vi "S2DS_ConfigWrite sweep info (SubVI).vi"(8 "error in (no error)":errorcluster, 9 "WC Channel names":string[](array[string]), 10 "Scan parameters in":T2 {"Y data taking" items=["in both direction", "in up direction only", "in down direction only"]; "X data taking" items=["in both direction", "in up direction only", "in down direction only"]}, 11 "Refnum in":T1) -> (0 "error out":errorcluster, 3 "Refnum out":T1)   [LabVIEW 2025]
uses:
  TYPE DEFS/S2DS_Sweep Info.ctl
  <vilib>/Utility/config.llb/Config Data RefNum.ctl
  <vilib>/Utility/config.llb/Write Key (String).vi
  <vilib>/Utility/config.llb/Write Key (I32).vi
  <vilib>/Utility/config.llb/Write Key (Double).vi
  <vilib>/Utility/config.llb/Write Key (U32).vi
  <vilib>/Utility/config.llb/Write Key (Boolean).vi
  <vilib>/Utility/config.llb/NI_LVConfig.lvlib
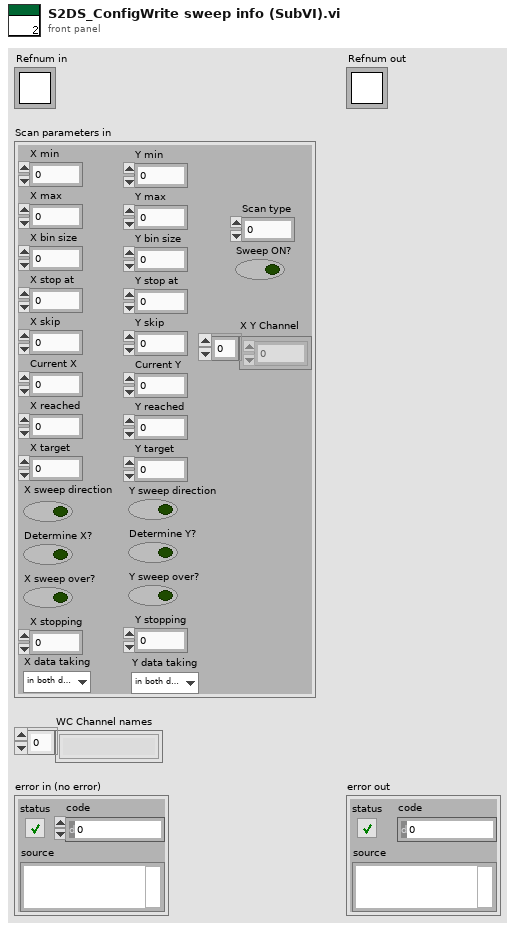
[diagram p1: front panel]
types:
  T1 = typedef "NI_LVConfig.lvlib/Config Data RefNum.ctl" = refnum<k1>
  T2 = typedef "S2DS_Sweep Info.ctl" = cluster{"X min":ext, "X max":dbl, "Y min":dbl, "Y max":dbl, "X bin size":dbl, "Y bin size":dbl, "X stop at":dbl, "Y stop at":dbl, "X skip":u64, "Y skip":u64, "Current X":dbl, "Current Y":dbl, "X reached":i32, "Y reached":i32, "X target":dbl, "Y target":dbl, "Sweep ON?":bool, "X sweep direction":bool, "Y sweep direction":bool, "Determine X?":bool, "Determine Y?":bool, "X sweep over?":bool, "Y sweep over?":bool, "Scan type":i32, "X stopping":i32, "Y stopping":i32, "X Y Channel":u16[], "X data taking":u16, "Y data taking":u16}
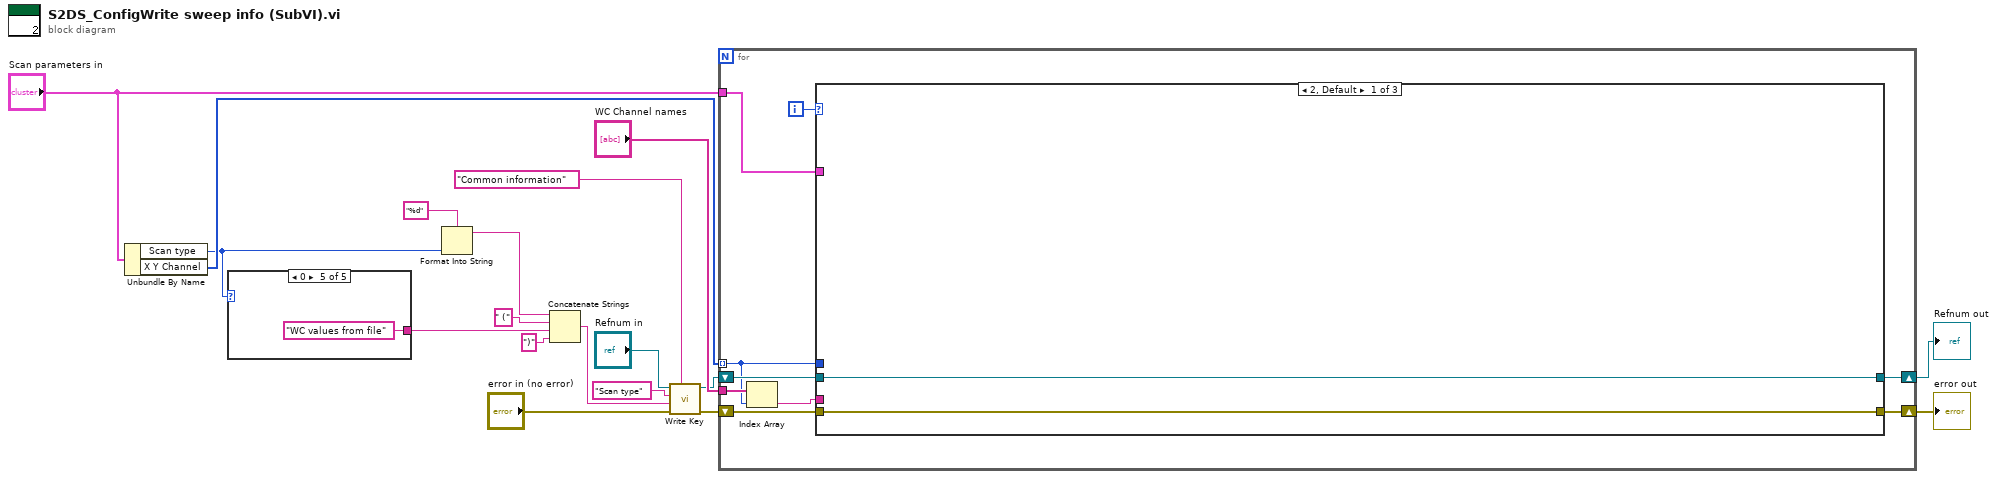
[diagram p0: block diagram]
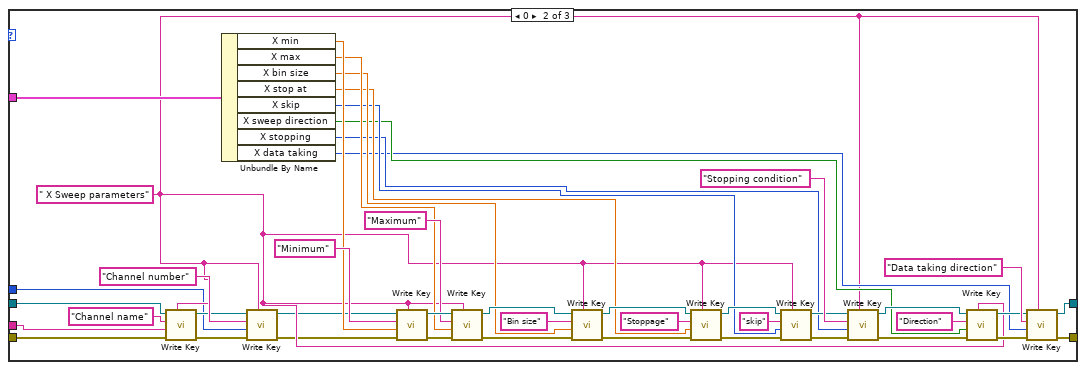
[diagram p2: hidden frame]
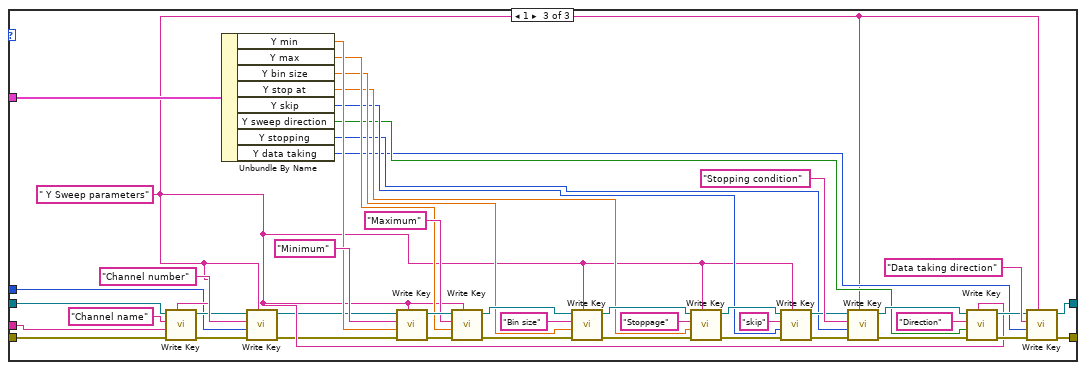
[diagram p3: hidden frame]
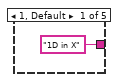
[diagram p4: hidden frame]
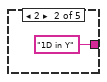
[diagram p5: hidden frame]
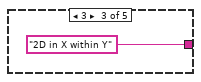
[diagram p6: hidden frame]
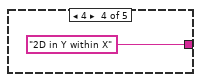
[diagram p7: hidden frame]
diagram:
  n1 = Unbundle By Name("Scan parameters in") -> ("Scan type"=w7:i32, "X Y Channel"=w10:u16[])
  n2 = case shown="0" w7 {
    tunnel: ["1D in X" "1D in Y" "2D in X within Y" "2D in Y within X" "WC values from file"] -> w2
    frame 1, Default {
    }
    frame 2 {
    }
    frame 3 {
    }
    frame 4 {
    }
    frame 0 {
    }
  }
  n3 = Format Into String(format string="%d", w7) -> (resulting string=w5:string)  [unwired: 2 in, 1 out]
  n4 = Concatenate Strings(w5, " (" ("string"), w2, ")" ("string")) -> (w1:string)
  n5 = call-poly <vilib>:"Write Key.vi"("section"="Common information", "error in (no error)"="error in (no error)", "value"=w1, "key"="Scan type", "refnum"="Refnum in") -> ("error out"=w12:errorcluster, "refnum out"=w11:T1)  [unwired: 4 in, 1 out]
  n6 = for {
    tunnel: w10 -> [w24] mode=indexing
    tunnel: "WC Channel names" -> [w32]
    shift-right: [w28] -> w14
    shift-left: w11 -> [w29]
    shift-right: [w27] -> w15
    shift-left: w12 -> [w30]
    tunnel: "Scan parameters in" -> [w31]
    i -> [w26]
    n7 = Index Array(array=w32, index=w24) -> (element=w25:string)
    n8 = case shown="2, Default" w26 {
      tunnel: w31 -> [_ w71 w115]
      tunnel: [w34 w47 w91] -> w28
      tunnel: [w33 w48 w92] -> w27
      tunnel: w29 -> [w34 w38 w82]
      tunnel: w30 -> [w33 w36 w80]
      tunnel: w25 -> [_ w44 w88]
      tunnel: w24 -> [_ w39 w83]
      frame 2, Default {
      }
      frame 0 {
        w41 = " X Sweep parameters"
        n9 = call-poly <vilib>:"Write Key.vi"("section"=w41, "error in (no error)"=w36, "value"=w44, "key"="Channel name", "refnum"=w38) -> ("error out"=w40:errorcluster, "refnum out"=w42:T1)  [unwired: 4 in, 1 out]
        n10 = Unbundle By Name(w71) -> ("X min"=w70:ext, "X max"=w69:dbl, "X bin size"=w68:dbl, "X stop at"=w55:dbl, "X skip"=w54:u64, "X sweep direction"=w53:bool, "X stopping"=w52:i32, "X data taking"=w46:u16)
        n11 = call-poly <vilib>:"Write Key.vi"("section"=w41, "error in (no error)"=w40, "value"=w39, "key"="Channel number", "refnum"=w42) -> ("error out"=w35:errorcluster, "refnum out"=w37:T1)  [unwired: 4 in, 1 out]
        n12 = call-poly <vilib>:"Write Key.vi"("section"=w41, "error in (no error)"=w35, "value"=w70, "key"="Minimum", "refnum"=w37) -> ("error out"=w77:errorcluster, "refnum out"=w75:T1)  [unwired: 4 in, 1 out]
        n13 = call-poly <vilib>:"Write Key.vi"("section"=w41, "error in (no error)"=w77, "value"=w69, "key"="Maximum", "refnum"=w75) -> ("error out"=w78:errorcluster, "refnum out"=w76:T1)  [unwired: 4 in, 1 out]
        n14 = call-poly <vilib>:"Write Key.vi"("section"=w41, "error in (no error)"=w78, "value"=w68, "key"="Bin size", "refnum"=w76) -> ("error out"=w56:errorcluster, "refnum out"=w57:T1)  [unwired: 4 in, 1 out]
        n15 = call-poly <vilib>:"Write Key.vi"("section"=w41, "error in (no error)"=w56, "value"=w55, "key"="Stoppage", "refnum"=w57) -> ("error out"=w60:errorcluster, "refnum out"=w63:T1)  [unwired: 4 in, 1 out]
        n16 = call-poly <vilib>:"Write Key.vi"("section"=w41, "error in (no error)"=w60, "value"=w54, "key"="skip", "refnum"=w63) -> ("error out"=w59:errorcluster, "refnum out"=w62:T1)  [unwired: 4 in, 1 out]
        n17 = call-poly <vilib>:"Write Key.vi"("section"=w41, "error in (no error)"=w59, "value"=w52, "key"="Stopping condition", "refnum"=w62) -> ("error out"=w58:errorcluster, "refnum out"=w61:T1)  [unwired: 4 in, 1 out]
        n18 = call-poly <vilib>:"Write Key.vi"("section"=w41, "error in (no error)"=w58, "value"=w53, "key"="Direction", "refnum"=w61) -> ("error out"=w49:errorcluster, "refnum out"=w50:T1)  [unwired: 4 in, 1 out]
        n19 = call-poly <vilib>:"Write Key.vi"("section"=w41, "error in (no error)"=w49, "value"=w46, "key"="Data taking direction", "refnum"=w50) -> ("error out"=w48:errorcluster, "refnum out"=w47:T1)  [unwired: 4 in, 1 out]
      }
      frame 1 {
        w85 = " Y Sweep parameters"
        n20 = call-poly <vilib>:"Write Key.vi"("section"=w85, "error in (no error)"=w80, "value"=w88, "key"="Channel name", "refnum"=w82) -> ("error out"=w84:errorcluster, "refnum out"=w86:T1)  [unwired: 4 in, 1 out]
        n21 = Unbundle By Name(w115) -> ("Y min"=w114:dbl, "Y max"=w113:dbl, "Y bin size"=w112:dbl, "Y stop at"=w99:dbl, "Y skip"=w98:u64, "Y sweep direction"=w97:bool, "Y stopping"=w96:i32, "Y data taking"=w90:u16)
        n22 = call-poly <vilib>:"Write Key.vi"("section"=w85, "error in (no error)"=w84, "value"=w83, "key"="Channel number", "refnum"=w86) -> ("error out"=w79:errorcluster, "refnum out"=w81:T1)  [unwired: 4 in, 1 out]
        n23 = call-poly <vilib>:"Write Key.vi"("section"=w85, "error in (no error)"=w79, "value"=w114, "key"="Minimum", "refnum"=w81) -> ("error out"=w121:errorcluster, "refnum out"=w119:T1)  [unwired: 4 in, 1 out]
        n24 = call-poly <vilib>:"Write Key.vi"("section"=w85, "error in (no error)"=w121, "value"=w113, "key"="Maximum", "refnum"=w119) -> ("error out"=w122:errorcluster, "refnum out"=w120:T1)  [unwired: 4 in, 1 out]
        n25 = call-poly <vilib>:"Write Key.vi"("section"=w85, "error in (no error)"=w122, "value"=w112, "key"="Bin size", "refnum"=w120) -> ("error out"=w100:errorcluster, "refnum out"=w101:T1)  [unwired: 4 in, 1 out]
        n26 = call-poly <vilib>:"Write Key.vi"("section"=w85, "error in (no error)"=w100, "value"=w99, "key"="Stoppage", "refnum"=w101) -> ("error out"=w104:errorcluster, "refnum out"=w107:T1)  [unwired: 4 in, 1 out]
        n27 = call-poly <vilib>:"Write Key.vi"("section"=w85, "error in (no error)"=w104, "value"=w98, "key"="skip", "refnum"=w107) -> ("error out"=w103:errorcluster, "refnum out"=w106:T1)  [unwired: 4 in, 1 out]
        n28 = call-poly <vilib>:"Write Key.vi"("section"=w85, "error in (no error)"=w103, "value"=w96, "key"="Stopping condition", "refnum"=w106) -> ("error out"=w102:errorcluster, "refnum out"=w105:T1)  [unwired: 4 in, 1 out]
        n29 = call-poly <vilib>:"Write Key.vi"("section"=w85, "error in (no error)"=w102, "value"=w97, "key"="Direction", "refnum"=w105) -> ("error out"=w93:errorcluster, "refnum out"=w94:T1)  [unwired: 4 in, 1 out]
        n30 = call-poly <vilib>:"Write Key.vi"("section"=w85, "error in (no error)"=w93, "value"=w90, "key"="Data taking direction", "refnum"=w94) -> ("error out"=w92:errorcluster, "refnum out"=w91:T1)  [unwired: 4 in, 1 out]
      }
    }
  }
  "error out" <- w15
  "Refnum out" <- w14
